vi "ArduinoLT-FULL-LightSwitch_and_TempMonitor-V2.vi"(8 "error in":errorcluster, 10 "Spotlights":bool, 11 "Coaxial light":bool) -> (0 "error out":errorcluster)   [LabVIEW 2016]
uses:
  <vilib>/LabVIEW Interface for Arduino/LabVIEW Interface for Arduino.lvlib
panel:
  out "Temperature Chart":dbl(graph)
  in  "stop":bool
  out "Loop Number":i32
  in  "VISA resource":refnum<visa-resource-name>="LightsCTRL"
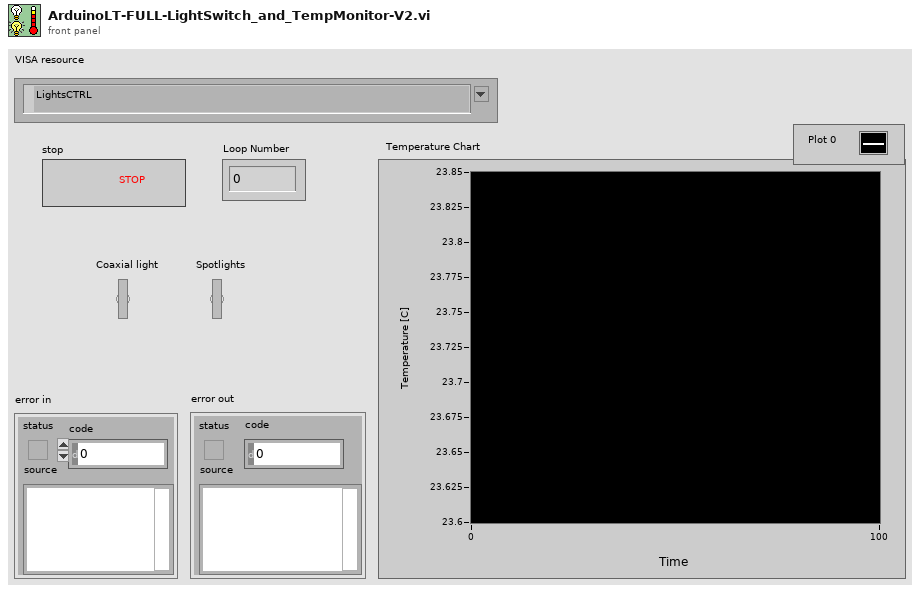
[diagram p1: front panel]
types:
  T1 = typedef "LabVIEW Interface for Arduino.lvlib/Arduino Resource.ctl" = cluster{"VISA resource":refnum<visa-resource-name>, "Board Type":T2, "Connection Type":enum8{"USB / Serial"}, "Bytes Per Packet (15)":u8}
  T2 = typedef "LabVIEW Interface for Arduino.lvlib/Board Type.ctl" = enum16{"Uno", "Dimuelanove w/Atmega 328", "Mega 2560"}
  T3 = typedef "ArduinoLT-ConfigurationControl.ctl" = cluster{"Lights: Digital I/O Pins":cluster{"Coaxial":u8, "Spotlights":u8}, "Thermistor Settings":cluster{"Analogue Readout Pin":u8, "Vcc Reference Pin":u8, "Paired Resistance (10K Ohms)":dbl, "Units (C)":enum16{"Celsius", "Fahrenheit", "Kelvin"}}}
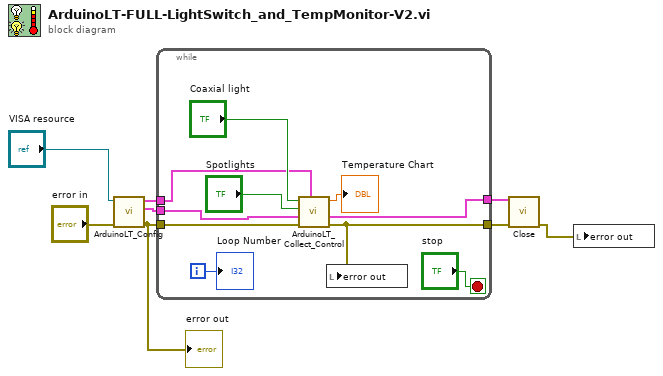
[diagram p0: block diagram]
diagram:
  n1 = call "ArduinoLT_Config.vi"("error in"="error in", "VISA resource"="VISA resource") -> ("error out"=w3:errorcluster, "Arduino Resource"=w1:T1, "Arduino Configuration OUT"=w7:T3)  [unwired: 3 in, 1 out]
  "error out" <- w3
  n2 = while {
    tunnel: w7 -> [w10]
    tunnel: w3 -> [w13]
    tunnel: [w12] -> w5
    tunnel: [w11] -> w4
    tunnel: w1 -> [w9]
    i -> [w18]
    stop <- "stop" stop-if-true
    n3 = call "ArduinoLT_Collect_Control.vi"("Arduino Configuration"=w10, "error in"=w13, "Arduino Resource IN"=w9, "Spotlights"="Spotlights", "Coaxial light"="Coaxial light") -> ("error out"=w11:errorcluster, "Arduino Resource OUT"=w12:T1, "Thermometer [C]"=→"Temperature Chart":dbl)  [unwired: 4 in]
    n4 = local write "error out"(w11) -> ()
    "Loop Number" <- w18
  }
  n5 = call <vilib>:"Close.vi"("Arduino Resource"=w5, "error in"=w4) -> ("error out"=w2:errorcluster)  [unwired: 13 in]
  n6 = local write "error out"(w2) -> ()
